vi "getUserEvent.vi"(8 "error in (no error)":errorcluster, 11 "StatisticsDisplay in":refnum<class "StatisticsDisplay.lvclass">) -> (0 "error out":errorcluster, 2 "user event":refnum<user-event>, 3 "StatisticsDisplay out":refnum<class "StatisticsDisplay.lvclass">)   [LabVIEW 2017, in "StatisticsDisplay.lvclass"]
uses:
  StatisticsDisplay.lvclass
  Observer/Observer.lvclass
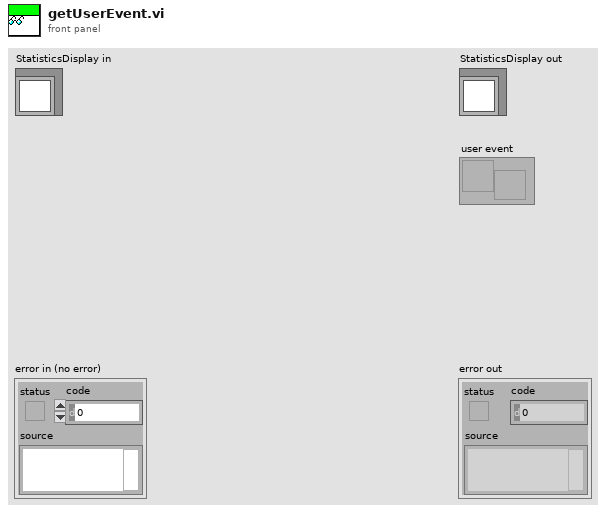
[diagram p1: front panel]
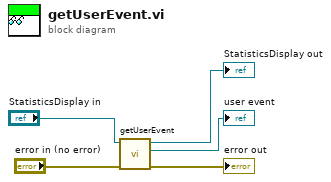
[diagram p0: block diagram]
diagram:
  n1 = call-parent "getUserEvent.vi"("error in (no error)"="error in (no error)", "Observer in"="StatisticsDisplay in") -> ("error out"=→"error out":errorcluster, "user event"=→"user event":refnum<user-event>, "Observer out"=→"StatisticsDisplay out":refnum<class "StatisticsDisplay.lvclass">)  [unwired: 7 in]
